vi "Perform Temp Test.vi"(8 "error in (no error)":errorcluster, 11 "LCM Single-Up MTS Test in":refnum<class "LCM Single-Up MTS Test.lvclass">) -> (0 "error out":errorcluster, 3 "Temperature Test Passed":bool)   [LabVIEW 2015, in "LCM Single-Up MTS Test.lvclass"]
uses:
  LCM Single-Up MTS Test.lvclass
  Classes/Instruments/Temperature Device/ThorLabs TSP01/Class/ThorLabs TSP01.lvclass
  Classes/Manufacturing Test/Class/SC Manufacturing Test.lvclass
  Classes/Test Recipe/Class/Test Recipe.lvclass
  Test Class/Test Class.lvclass
  Classes/Application/Class/Application.lvclass
  <vilib>/Cree, Inc/Cree Test Framework/Classes/Base Objects/Base Class/Base Class/Base Class.lvclass
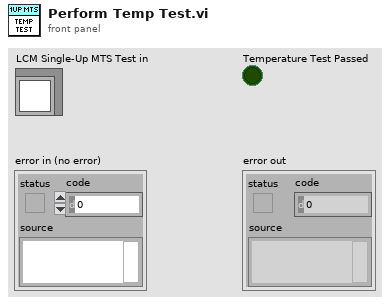
[diagram p1: front panel]
types:
  T1 = typedef "Application.lvlib/App Properties.lvclass/Class Properties -- Cluster.ctl" = cluster{"UUT Info":T2[], "Test Information":refnum<vi>, "Test Complete Event":refnum<user-event>, "Shop Floor System":refnum<class "Shop Floor System.lvclass">, "Gold Board":refnum<class "Golden Board.lvclass">, "Test Recipe":refnum<class "Test Recipe.lvclass">, "Instruments":refnum<class "Instrument.lvclass">[], "Mode":T3, "Test Results":cluster{"Pass":bool[], "Fail Codes":string[]}, "Station Config":refnum<class "Station Config.lvclass">}
  T2 = typedef "Application.lvlib/App Properties.lvclass/UUT Reference -- Cluster.ctl" = cluster{"Serial Number Reference":refnum<vi>, "Status Message Reference":refnum<vi>}
  T3 = typedef "Application.lvlib/Application.lvclass/Op Mode -- Enum.ctl" = u16
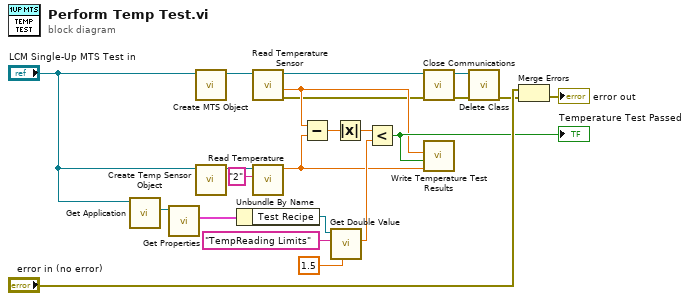
[diagram p0: block diagram]
diagram:
  n1 = call "Get Application.vi"("Test Class in"="LCM Single-Up MTS Test in") -> ("Application.lvlib:Application.lvclass"=w12:refnum<class "Application.lvclass">)  [unwired: 9 in, 1 out]
  n2 = call "Get Properties.vi"("Acrobat Template in"=w12) -> ("Class Properties"=w11:T1)  [unwired: 8 in, 2 out]
  n3 = call "Create MTS Object.vi"("LCM Single-Up MTS Test in"="LCM Single-Up MTS Test in") -> ("MTS"=w13:refnum<class "SC Manufacturing Test.lvclass">)  [unwired: 9 in, 1 out]
  n4 = call "Create Temp Sensor Object.vi"("LCM Single-Up MTS Test in"="LCM Single-Up MTS Test in") -> ("ThorLabs TSP01 out"=w7:refnum<class "ThorLabs TSP01.lvclass">)  [unwired: 9 in, 1 out]
  n5 = Unbundle By Name(w11) -> ("Test Recipe"=w9:refnum<class "Test Recipe.lvclass">)
  n6 = call "Read Temperature Sensor.vi"("Acrobat Template in"=w13) -> ("error out"=w2:errorcluster, "Temperature"=w8:dbl, "Acrobat Template out"=w4:refnum<class "SC Manufacturing Test.lvclass">)  [unwired: 8 in]
  n7 = call-dynamic "Read Temperature.vi"("Channel"="2", "Acrobat Template in"=w7) -> ("Temperature out"=w5:dbl)  [unwired: 8 in, 1 out]
  n8 = Subtract(x=w8, y=w5) -> (x-y=w15:dbl)
  n9 = call "Get Double Value.vi"("Default Value"=1.5, "Name"="TempReading Limits", "Test Recipe in"=w9) -> ("Value"=w17:dbl)  [unwired: 6 in, 2 out]
  n10 = Absolute Value(x=w15) -> (abs(x)=w16:dbl)
  n11 = Less?(x=w16, y=w17) -> (x < y?=w20:bool)
  "Temperature Test Passed" <- w20
  n12 = call "Close Communications.vi"("error in (no error)"=w2, "Acrobat Template in"=w4) -> ("error out"=w1:errorcluster, "Acrobat Template out"=w3:refnum<class "SC Manufacturing Test.lvclass">)  [unwired: 8 in]
  n13 = call "Write Temperature Test Results.vi"("Actual Temperature"=w5, "Pass Fail"=w20, "MTS Temperature"=w8) -> ()  [unwired: 9 in]
  n14 = call <vilib>:"Delete Class.vi"("error in (no error)"=w1, "Base Class in"=w3) -> ("error out"=w19:errorcluster)  [unwired: 8 in, 1 out]
  n15 = Merge Errors("error in (no error)", w19) -> (→"error out":errorcluster)
